vi "Handshake.vi"(8 "error in (no error)":errorcluster, 10 "Request":refnum<class "Request.lvclass">) -> (0 "error out":errorcluster, 1 "Response out":refnum<class "WebSocketUpgradeResponse.lvclass">, 2 "Is WS Upgrade":bool)   [LabVIEW 2020, in "HTTP Server.lvlib" / "WebSocket Client.lvclass"]
uses:
  WebSocket Client.lvclass
  WebSocketUpgradeResponse/WebSocketUpgradeResponse.lvclass
  WebSocket Client.lvclass/WebSocket Client.ctl
  lv-http-util/HTTP Utils/Request/Request.lvclass
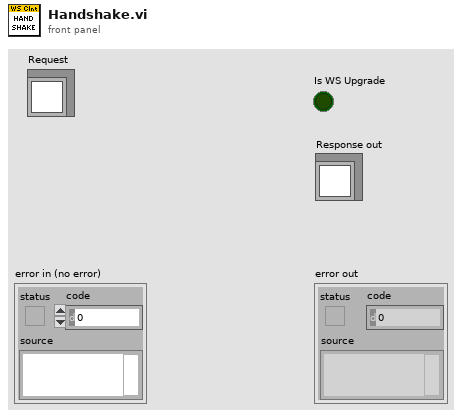
[diagram p1: front panel]
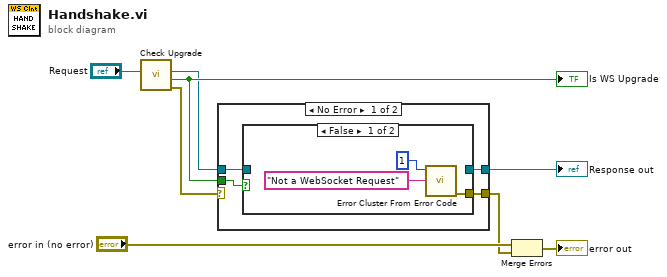
[diagram p0: block diagram]
diagram:
  n1 = call "Check Upgrade.vi"("Request"="Request") -> ("error out"=w7:errorcluster, "Is WS Upgrade"=w6:bool, "Response"=w5:refnum<class "WebSocketUpgradeResponse.lvclass">)  [unwired: 8 in]
  "Is WS Upgrade" <- w6
  n2 = case shown="No Error" w7 {
    selector: w7 -> [_ w17]
    tunnel: w6 -> [w12 _]
    tunnel: w5 -> [w11 _]
    tunnel: [w10 w17] -> w3
    tunnel: [w9 _] -> w2
    frame No Error {
      n3 = case shown="False" w12 {
        tunnel: w11 -> [_ w16]
        tunnel: [w13 _] -> w10
        tunnel: [_ w16] -> w9
        frame False {
          n4 = call <vilib>:"Error Cluster From Error Code.vi"("error message (\"\")"="Not a WebSocket Request" ("error message (\"\")"), "error code (0)"=1) -> ("error out"=w13:errorcluster)  [unwired: 7 in]
        }
        frame True {
        }
      }
    }
    frame Error {
    }
  }
  "Response out" <- w2
  n5 = Merge Errors("error in (no error)", w3) -> (→"error out":errorcluster)
